vi "SplitFilterOutput.vi"(11 "filter output":fxp<+,64,64>) -> (2 "Q out":fxp<+/-,16,14>, 3 "I out":fxp<+/-,16,14>)   [LabVIEW 2013]
uses:
  <vilib>/rvi/FXPMathLib/FxpConvert/subVIs/nifxpmath_Convert_SimConfig.ctl
  <vilib>/fxp/LVFixedPointQuantizationPolicyTypeDef.ctl
  <vilib>/fxp/LVFixedPointOverflowPolicyTypeDef.ctl
  <vilib>/rvi/FXPMathLib/FxpConvert/simVIs/DllFxpConvertTemp_sub.vi
  <vilib>/rvi/FXPMathLib/FxpInterpret/XNode/nifxpmath_Interpret.xnode
  <vilib>/rvi/FXPMathLib/FxpConvert/XNode/nifxpmath_Convert.xnode
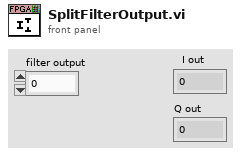
[diagram p1: front panel]
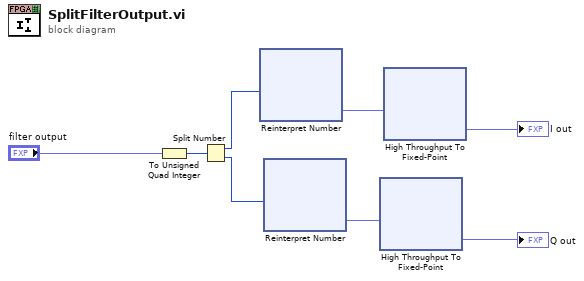
[diagram p0: block diagram]
diagram:
  n1 = To Unsigned Quad Integer(1:"filter output") -> (0:w7:u64)
  n2 = Split Number(x=w7) -> (hi(x)=w8:u32, lo(x)=w1:u32)
  n3 = xnode "Reinterpret Number"("x"=w8) -> ("y"=w4:fxp<+/-,32,15>)
  n4 = xnode "Reinterpret Number"("x"=w1) -> ("y"=w6:fxp<+/-,32,15>)
  n5 = xnode "High Throughput To Fixed-Point"("x"=w6) -> ("y"=→"Q out":fxp<+/-,16,14>)
  n6 = xnode "High Throughput To Fixed-Point"("x"=w4) -> ("y"=→"I out":fxp<+/-,16,14>)
